vi "GetProperties.vi"(8 "error in":errorcluster, 11 "Generic in":refnum<class "Generic.lvclass">) -> (0 "error out":errorcluster, 3 "Generic out":refnum<class "Generic.lvclass">)   [LabVIEW 2014, in "Generic.lvclass"]
uses:
  Generic.lvclass
  Generic.lvclass/Generic.ctl
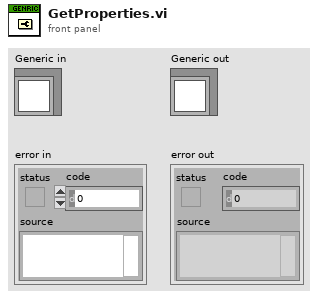
[diagram p1: front panel]
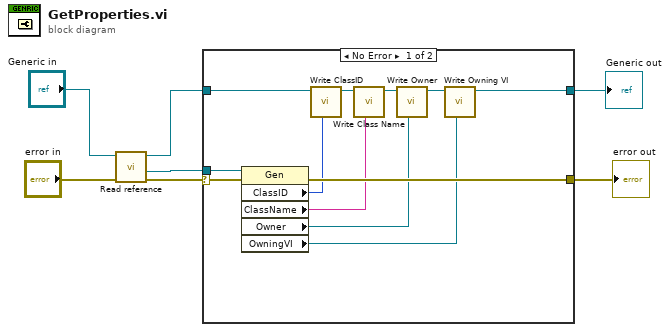
[diagram p0: block diagram]
diagram:
  n1 = call "Read reference.vi"("error in"="error in", "GObject in"="Generic in") -> ("error out"=w2:errorcluster, "reference"=w3:refnum<vi>, "GObject out"=w4:refnum<class "Generic.lvclass">)  [unwired: 5 in]
  n2 = case shown="No Error" w2 {
    selector: w2 -> [w18 w20]
    tunnel: w3 -> [w19 _]
    tunnel: w4 -> [w8 w21]
    tunnel: [w9 w21] -> w7
    tunnel: [w17 w20] -> w6
    frame No Error {
      n3 = property class="Gen"(reference=w19, error in=w18) -> (error out=w17:errorcluster, "ClassID"=w16:u32, "ClassName"=w14:string, "Owner"=w12:refnum<vi>, "OwningVI"=w10:refnum<vi>)  [unwired: 1 out]
      n4 = call "Write ClassID.vi"("ClassID"=w16, "Generic in"=w8) -> ("Generic out"=w15:refnum<class "Generic.lvclass">)  [unwired: 7 in]
      n5 = call "Write Class Name.vi"("Class Name"=w14, "Generic in"=w15) -> ("Generic out"=w13:refnum<class "Generic.lvclass">)  [unwired: 7 in]
      n6 = call "Write Owner.vi"("Owner"=w12, "Generic in"=w13) -> ("Generic out"=w11:refnum<class "Generic.lvclass">)  [unwired: 7 in]
      n7 = call "Write Owning VI.vi"("Owning VI"=w10, "Generic in"=w11) -> ("Generic out"=w9:refnum<class "Generic.lvclass">)  [unwired: 7 in]
    }
    frame Error {
    }
  }
  "error out" <- w6
  "Generic out" <- w7
